vi "VI Tree.vi"   [LabVIEW 2012, in "Phidget Current Input.lvlib"]
doc: "${CurrentInput:VITreeHeader}"
uses:
  <instrlib>/Phidgets/Phidget Current Input/Phidget Current Input.lvlib
  <instrlib>/Phidgets/Phidget Current Input/Public/CurrentInputStart.vi
  <instrlib>/Phidgets/Phidget Current Input/Public/CurrentInputOpen.vi
  <instrlib>/Phidgets/Phidget Current Input/Public/CurrentInputClose.vi
panel:
  # "(c) 2015 Phidgets Inc..  ALL RIGHTS RESERVED."
  # "SEE DIAGRAM\nFOR VI TREE."
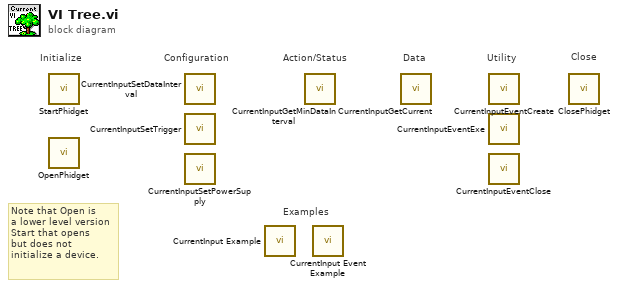
[diagram p0: block diagram]
diagram:
  # "Note that Open is\na lower level version\nStart that opens\nbut does not \ninitialize a device."
  # "Examples"
  # "Configuration"
  # "Utility"
  # "Data"
  # "Action/Status"
  # "Close"
  # "Initialize"
  n1 = call-poly <instrlib>:"StartPhidget.vi"() -> ()  [unwired: 12 in, 4 out]
  n2 = call-poly <instrlib>:"OpenPhidget.vi"() -> ()  [unwired: 8 in, 4 out]
  n3 = call <instrlib>:"CurrentInputSetDataInterval.vi"() -> ()  [unwired: 9 in, 2 out]
  n4 = call <instrlib>:"CurrentInputSetTrigger.vi"() -> ()  [unwired: 9 in, 2 out]
  n5 = call <instrlib>:"CurrentInputSetPowerSupply.vi"() -> ()  [unwired: 9 in, 2 out]
  n6 = call <instrlib>:"CurrentInput Example.vi"() -> ()  [unwired: 12 in]
  n7 = call <instrlib>:"CurrentInputGetMinDataInterval.vi"() -> ()  [unwired: 8 in, 3 out]
  n8 = call <instrlib>:"CurrentInput Event Example.vi"() -> ()  [unwired: 12 in]
  n9 = call <instrlib>:"CurrentInputGetCurrent.vi"() -> ()  [unwired: 8 in, 3 out]
  n10 = call <instrlib>:"CurrentInputEventCreate.vi"() -> ()  [unwired: 9 in, 3 out]
  n11 = call <instrlib>:"CurrentInputEventExe.vi"() -> ()  [unwired: 5 in, 7 out]
  n12 = call <instrlib>:"CurrentInputEventClose.vi"() -> ()  [unwired: 10 in, 2 out]
  n13 = call-poly <instrlib>:"ClosePhidget.vi"() -> ()  [unwired: 11 in, 1 out]
